vi "us read.vi"(8 "Error In":errorcluster, 11 "my FPGA lib.lvlib:US sensor.lvclass":refnum<class "US sensor.lvclass">) -> (0 "error out":errorcluster, 1 "timeout?":bool, 2 "distance(cm)":dbl, 3 "my FPGA lib.lvlib:US sensor.lvclass 2":refnum<class "US sensor.lvclass">)   [LabVIEW 2019, in "my FPGA lib.lvlib" / "US sensor.lvclass"]
uses:
  US sensor.lvclass
  US sensor.lvclass/US sensor.ctl
  <vilib>/Utility/error.llb/Error Cluster From Error Code.vi
  <vilib>/rvi/errors/niLvFpgaAdjustHostInterfaceError.vi
  <vilib>/rvi/interface/nirviReadWriteControl/nirviReadWriteControl.xnode
  NiFpgaLv.dll
  <vilib>/rvi/interface/Simulation/niFpgaSimulationCallBeginRW.vi
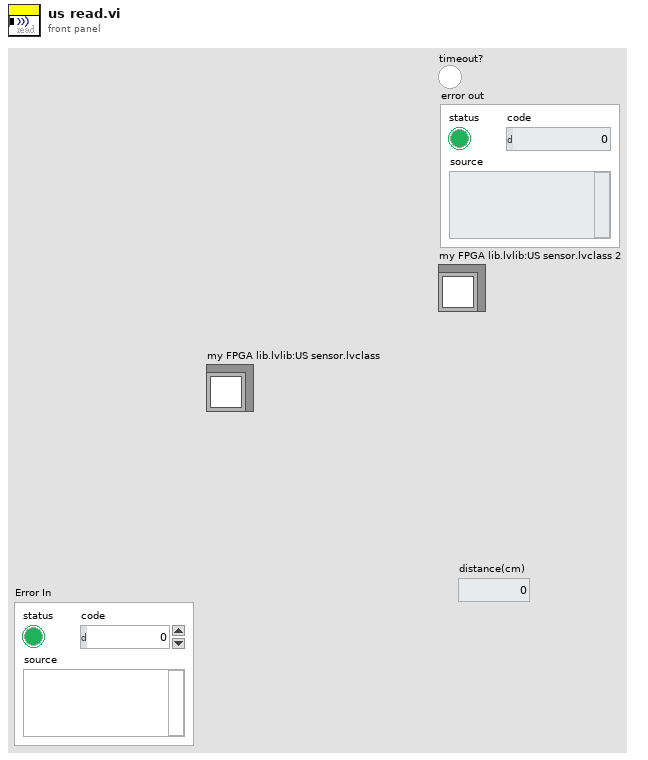
[diagram p1: front panel]
types:
  T1 = typedef "my FPGA lib.lvlib/US sensor.lvclass/us select.ctl" = enum16{"US.1", "US.2", "US.3", "US.4"}
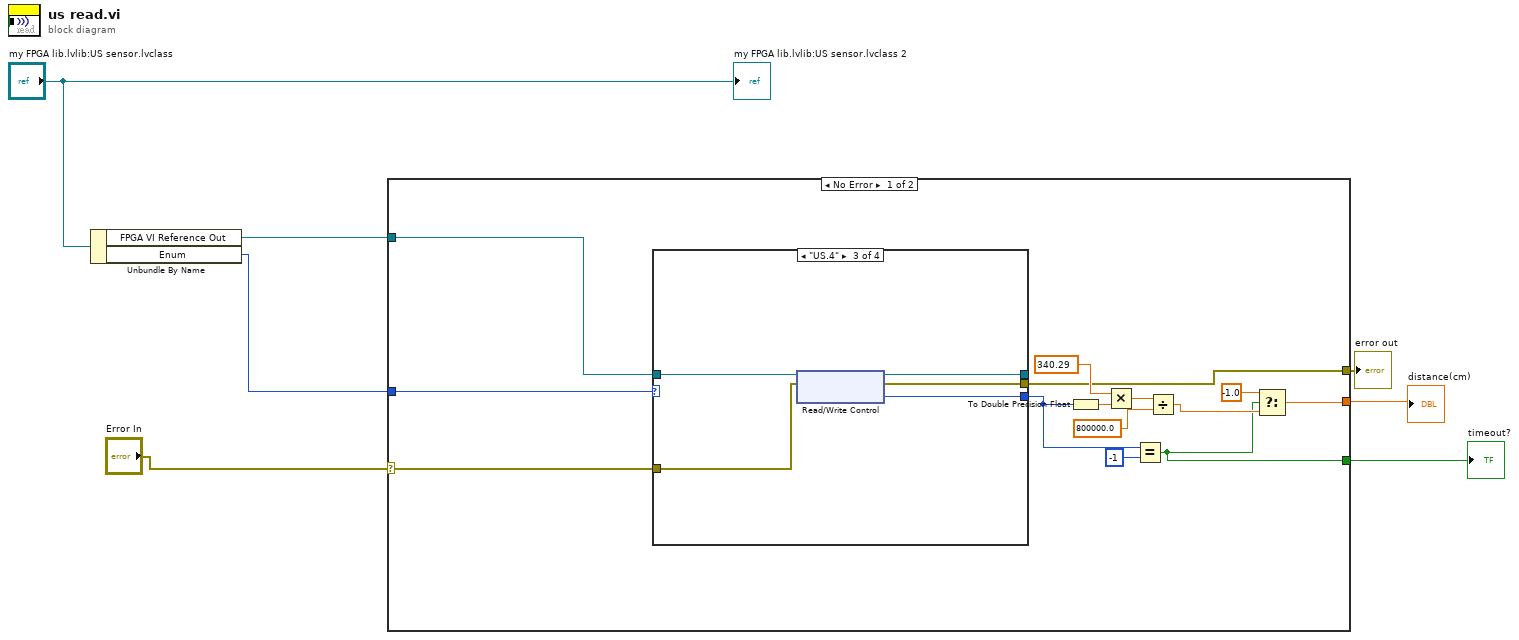
[diagram p0: block diagram]
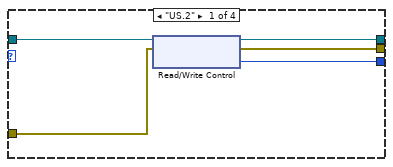
[diagram p2: hidden frame]
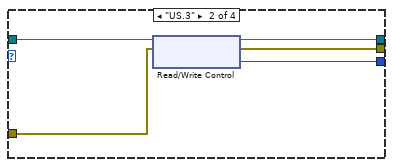
[diagram p3: hidden frame]
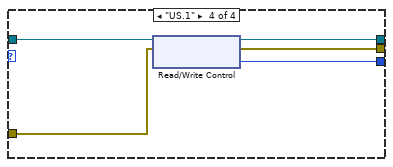
[diagram p4: hidden frame]
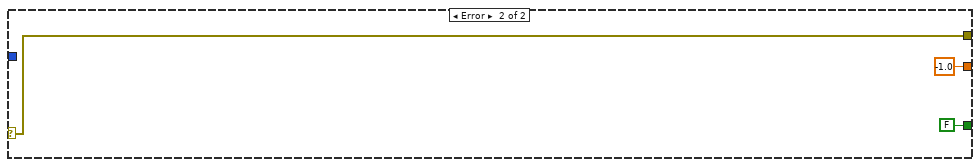
[diagram p5: hidden frame]
diagram:
  n1 = Unbundle By Name("my FPGA lib.lvlib:US sensor.lvclass") -> ("FPGA VI Reference Out"=w4:refnum<k20>, "Enum"=w6:T1)
  n2 = case shown="No Error" "Error In" {
    selector: "Error In" -> [w19 w42]
    tunnel: w6 -> [w21 _]
    tunnel: w4 -> [w20 _]
    tunnel: [w10 -1.0 ("t")] -> w3
    tunnel: [w9 FALSE] -> w2
    tunnel: [w8 w42] -> w1
    frame No Error {
      n3 = case shown="\"US.4\"" w21 {
        tunnel: w20 -> [w26 w31 w36 w41]
        tunnel: w19 -> [w25 w30 w35 w40]
        tunnel: [w24 w29 w34 w39] -> w8
        tunnel: [w23 w28 w33 w38] -> _
        tunnel: [w22 w27 w32 w37] -> w17
        frame "US.2" {
          n4 = xnode "Read/Write Control"("FPGA VI Reference In"=w26, "error in"=w25) -> ("FPGA VI Reference Out"=w23:refnum<k20>, "error out"=w24:errorcluster, "us2.distance"=w22:i32)
        }
        frame "US.3" {
          n5 = xnode "Read/Write Control"("FPGA VI Reference In"=w31, "error in"=w30) -> ("FPGA VI Reference Out"=w28:refnum<k20>, "error out"=w29:errorcluster, "us3.distance"=w27:i32)
        }
        frame "US.4" {
          n6 = xnode "Read/Write Control"("FPGA VI Reference In"=w36, "error in"=w35) -> ("FPGA VI Reference Out"=w33:refnum<k20>, "error out"=w34:errorcluster, "us4.distance"=w32:i32)
        }
        frame "US.1" {
          n7 = xnode "Read/Write Control"("FPGA VI Reference In"=w41, "error in"=w40) -> ("FPGA VI Reference Out"=w38:refnum<k20>, "error out"=w39:errorcluster, "us1.distance"=w37:i32)
        }
      }
      n8 = To Double Precision Float(number=w17) -> (double precision float=w16:dbl)
      n9 = Multiply(x=340.29, y=w16) -> (x*y=w14:dbl)
      n10 = Equal?(x=w17, y=-1) -> (x = y?=w9:bool)
      n11 = Divide(x=w14, y=800000.0) -> (x/y=w12:dbl)
      n12 = Select(t=-1.0, s=w9, f=w12) -> (s? t:f=w10:dbl)
    }
    frame Error {
    }
  }
  "distance(cm)" <- w3
  "timeout?" <- w2
  "error out" <- w1
  "my FPGA lib.lvlib:US sensor.lvclass 2" <- "my FPGA lib.lvlib:US sensor.lvclass"
